vi "GOOP_ShowHelp.vi"(0 "File":string) -> ()   [LabVIEW 2020]
uses:
  <vilib>/Platform/browser.llb/Open URL in Default Browser (path).vi
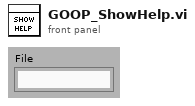
[diagram p1: front panel]
types:
  T1 = enum32{"invalid OS target", "Mac OS", "Windows 3.1", "Windows 95/NT", "Solaris 1", "Solaris 2", "HP-UX", "PowerMAX", "Linux", "Irix", "Rhapsody", "BeOS", "AIX", "OSF1", "VxWorks", "PharLap", "Carbon", "RTX", "Windows x64", "Linux x64"}
  T2 = enum32{"invalid OS target", "Mac OS", "Windows 3.1", "Windows 95/NT", "Solaris 1", "Solaris 2", "HP-UX", "PowerMAX", "Linux", "Irix", "Rhapsody", "BeOS", "AIX", "OSF1", "VxWorks", "PharLap", "Carbon", "RTX", "Windows x64", "Linux x64", "Mac OS X x64"}
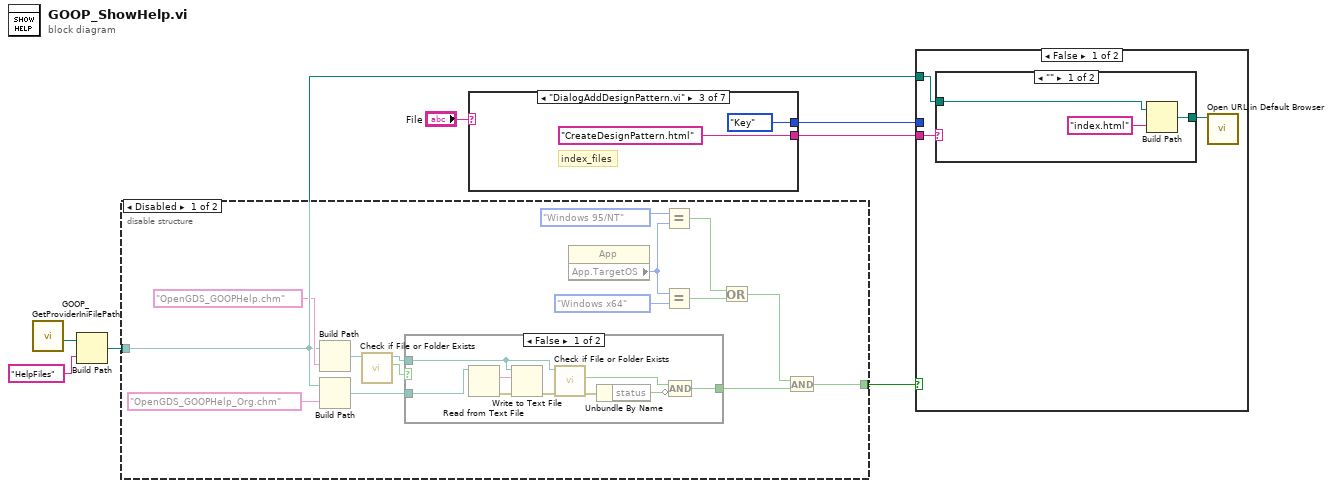
[diagram p0: block diagram]
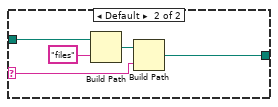
[diagram p4: hidden frame]
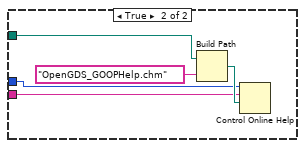
[diagram p5: hidden frame]
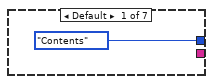
[diagram p6: hidden frame]
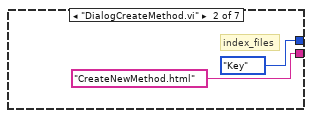
[diagram p7: hidden frame]
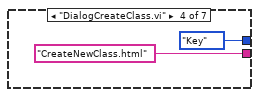
[diagram p8: hidden frame]
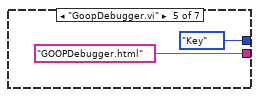
[diagram p9: hidden frame]
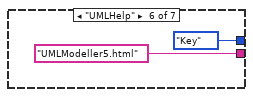
[diagram p10: hidden frame]
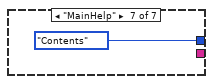
[diagram p11: hidden frame]
diagram:
  n1 = call "GOOP_GetProviderIniFilePath.vi"() -> ("ProviderMainFolder"=w1:path)  [unwired: 10 in, 1 out]
  n2 = Build Path(base path=w1, name or relative path="HelpFiles") -> (appended path=w3:path)
  n3 = disable-structure shown="Disabled" {
    disable-tunnel: w3 -> [w17 _]
    disable-tunnel: [w9 _] -> w2
    frame Disabled {
      n4 = Build Path(base path=w17, name or relative path="OpenGDS_GOOPHelp.chm") -> (appended path=w21:path)
      n5 = Build Path(base path=w17, name or relative path="OpenGDS_GOOPHelp_Org.chm") -> (appended path=w16:path)
      n6 = call <vilib>:"Check if File or Folder Exists.vi"("path"=w21) -> ("file or folder exists?"=w20:bool, "dup path"=w19:path)  [unwired: 8 in, 1 out]
      n7 = case shown="False" w20 {
        selector: w20 -> [_ w32]
        tunnel: [w23 w32] -> w8
        tunnel: w19 -> [w27 _]
        tunnel: w16 -> [w31 _]
        frame False {
          n8 = Read from Text File(file (use dialog)=w31) -> (text=w30:string, error out=w29:errorcluster)  [unwired: 3 in, 2 out]
          n9 = Write to Text File(file (use dialog)=w27, text=w30, error in=w29) -> (error out=w28:errorcluster)  [unwired: 1 in, 2 out]
          n10 = call <vilib>:"Check if File or Folder Exists.vi"("error in (no error)"=w28, "path"=w27) -> ("error out"=w25:errorcluster, "file or folder exists?"=w26:bool)  [unwired: 7 in, 1 out]
          n11 = Unbundle By Name(w25) -> ("status"=w24:bool)
          n12 = Compound Arithmetic op=AND(w26, invert w24) -> (w23:bool)
        }
        frame True {
        }
      }
      n13 = property class="App"() -> ("App.TargetOS"=w14:T2)  [unwired: 2 in, 2 out]
      n14 = Equal?(x=T1."Windows 95/NT" ("y"), y=w14) -> (x = y?=w12:bool)
      n15 = Equal?(x=w14, y=T1."Windows x64") -> (x = y?=w11:bool)
      n16 = Or(x=w12, y=w11) -> (x .or. y?=w10:bool)
      n17 = And(x=w10, y=w8) -> (x .and. y?=w9:bool)
    }
    frame Enabled {
    }
  }
  n18 = case shown="\"DialogAddDesignPattern.vi\"" "File" {
    tunnel: [_ "CreateNewMethod.html" "CreateDesignPattern.html" "CreateNewClass.html" "GOOPDebugger.html" "UMLModeller5.html" _] -> w5
    tunnel: [enum16{"Contents", "Key", "Close"}."Contents" ("Operation") enum16{"Contents", "Key", "Close"}."Key" ("Operation") enum16{"Contents", "Key", "Close"}."Key" ("Operation") enum16{"Contents", "Key", "Close"}."Key" ("Operation") enum16{"Contents", "Key", "Close"}."Key" ("Operation") enum16{"Contents", "Key", "Close"}."Key" ("Operation") enum16{"Contents", "Key", "Close"}."Contents" ("Operation")] -> w7
    frame Default {
    }
    frame "DialogCreateMethod.vi" {
      # "index_files"
    }
    frame "DialogAddDesignPattern.vi" {
      # "index_files"
    }
    frame "DialogCreateClass.vi" {
    }
    frame "GoopDebugger.vi" {
    }
    frame "UMLHelp" {
    }
    frame "MainHelp" {
    }
  }
  n19 = case shown="False" w2 {
    tunnel: w5 -> [w47 w56]
    tunnel: w3 -> [w45 w58]
    tunnel: w7 -> [_ w57]
    frame False {
      n20 = case shown="\"\"" w47 {
        selector: w47 -> [_ w54]
        tunnel: w45 -> [w50 w52]
        tunnel: [w49 w55] -> w46
        frame "" {
          n21 = Build Path(base path=w50, name or relative path="index.html") -> (appended path=w49:path)
        }
        frame Default {
          n22 = Build Path(base path=w52, name or relative path="files") -> (appended path=w51:path)
          n23 = Build Path(base path=w51, name or relative path=w54) -> (appended path=w55:path)
        }
      }
      n24 = call-poly <vilib>:"Open URL in Default Browser.vi"("path"=w46) -> ()  [unwired: 5 in, 2 out]
    }
    frame True {
      n25 = Build Path(base path=w58, name or relative path="OpenGDS_GOOPHelp.chm") -> (appended path=w60:path)
      n26 = Control Online Help(2:w60, 3:w56, 4:w57) -> ()  [unwired: 1 in, 1 out]
    }
  }
